vi "Save校准Spec.vi"(4 "补偿值":T3={"甩线补偿值"={"下边"=23.0, "距离上边"=10.0, "左边"=7.2, "右边"=25.8}, "补偿甩线坐标偏移"={"X"=40.0, "Y"=70.0}, "mark点补偿"={"X"=-48.38, "Y"=-84.85}, "出线补偿值"=25.8, "mark规格"={"X下限"=-48.0, "X上限"=-84.0, "Y下限"=0.0, "Y 上限"=0.0, "angle下限"=0.0, "angle上限"=0.0}} {"mark规格"."angle上限" format="%#.3f"; "mark规格"."angle下限" format="%#.3f"; "mark规格"."Y下限" format="%#.3f"; "mark规格"."X下限" format="%#.3f"; "mark点补偿"."X" format="%#.3f"; "补偿甩线坐标偏移"."X" format="%#.3f"}) -> ()   [LabVIEW 2014]
uses:
  Controls/XYPos.ctl
  Global.vi
  <vilib>/Utility/file.llb/Write To Spreadsheet File (string).vi
panel:
  out "数组":string[][](array[string])
  out "File out":path
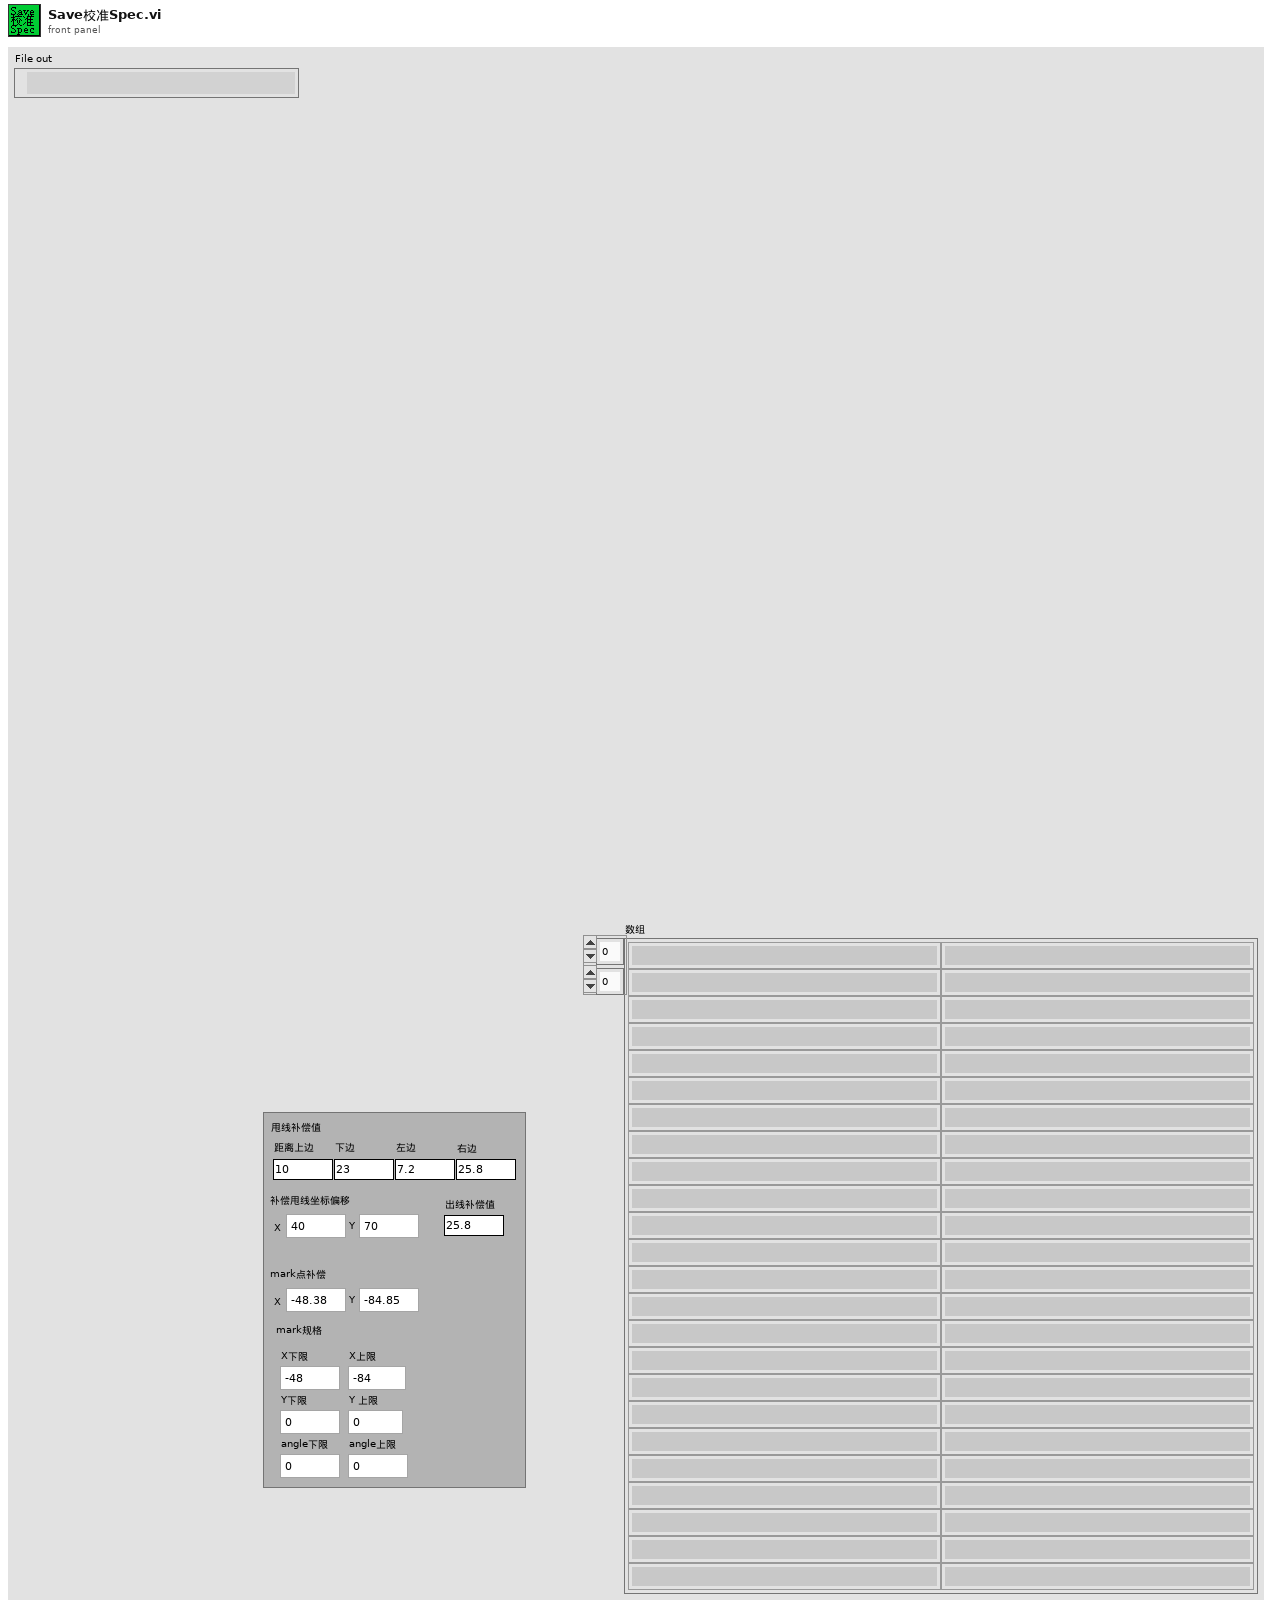
[diagram p1: front panel]
types:
  T1 = typedef "XYPos.ctl" = cluster{"X":dbl, "Y":dbl}
  T2 = typedef "mark规格.ctl" = cluster{"X下限":dbl, "X上限":dbl, "Y下限":dbl, "Y 上限":dbl, "angle下限":dbl, "angle上限":dbl}
  T3 = cluster{"甩线补偿值":cluster{"下边":dbl, "距离上边":dbl, "左边":dbl, "右边":dbl}, "补偿甩线坐标偏移":T1, "mark点补偿":T1, "出线补偿值":dbl, "mark规格":T2}
  T4 = cluster{"下边":dbl, "距离上边":dbl, "左边":dbl, "右边":dbl}
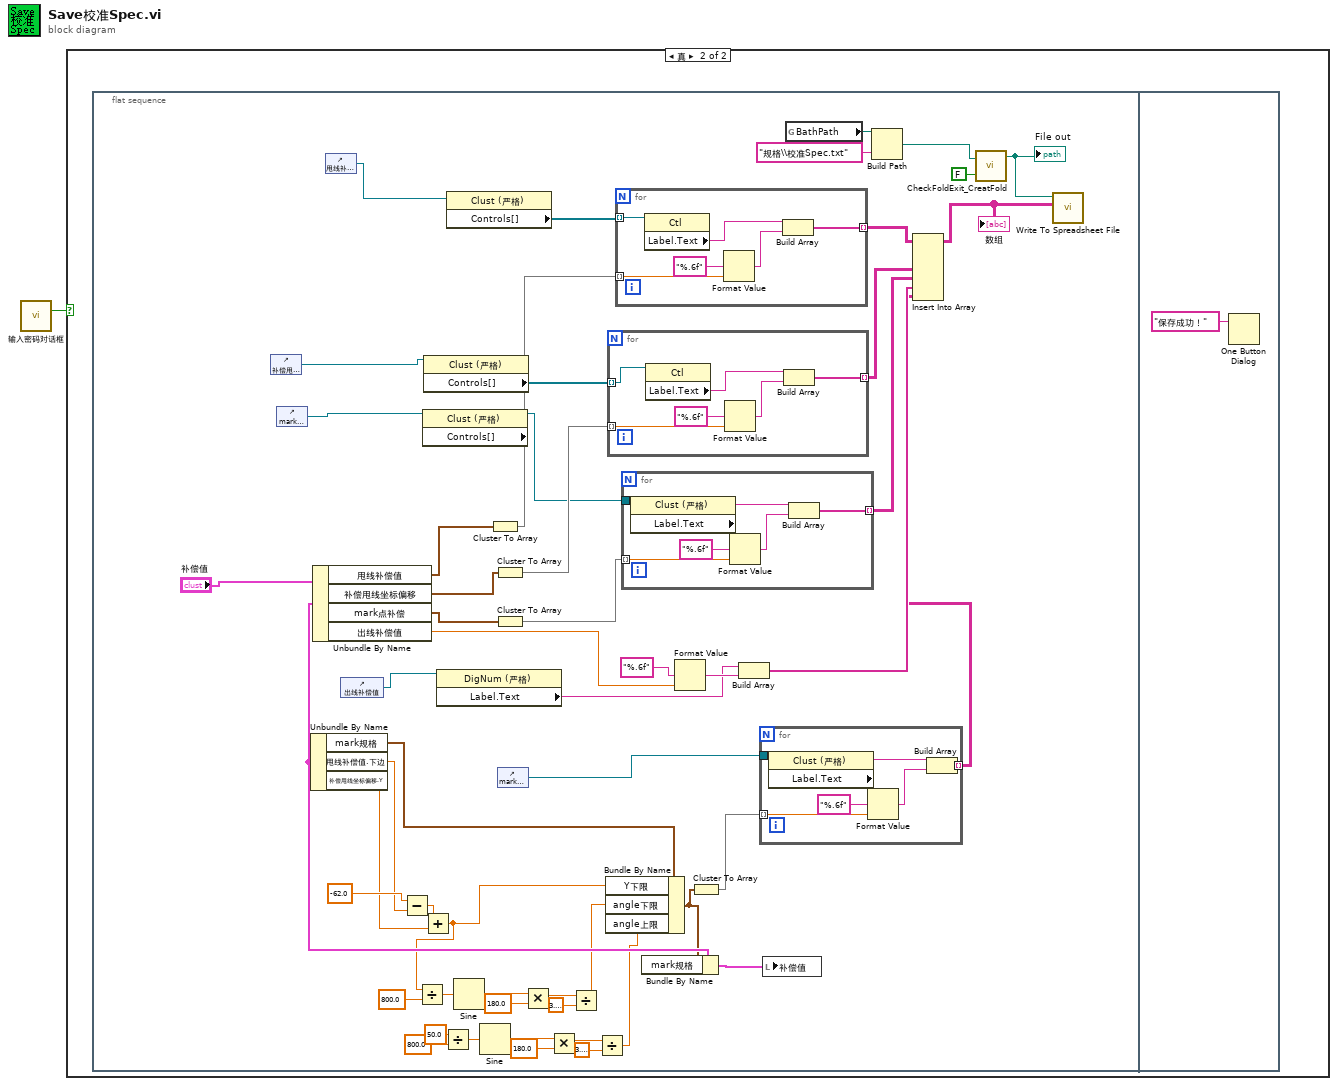
[diagram p0: block diagram]
diagram:
  n1 = call "输入密码对话框.vi"() -> ("密码正确"=w1:bool)  [unwired: 11 in]
  n2 = case shown="真" w1 {
    frame False {
    }
    frame True {
      n3 = flat-sequence {
        frame #0 {
          n4 = control-ref of="补偿甩线坐标偏移"() -> (w37:refnum<vi>)
          n5 = control-ref of="mark点补偿"() -> (w36:refnum<vi>)
          n6 = Unbundle By Name("补偿值") -> ("mark规格"=w23:T2, "甩线补偿值.下边"=w26:dbl, "补偿甩线坐标偏移.Y"=w24:dbl)
          n7 = Unbundle By Name("补偿值") -> ("甩线补偿值"=w27:T4, "补偿甩线坐标偏移"=w47:T1, "mark点补偿"=w45:T1, "出线补偿值"=w33:dbl)
          n8 = control-ref of="甩线补偿值"() -> (w38:refnum<vi>)
          n9 = control-ref of="出线补偿值"() -> (w35:refnum<vi>)
          n10 = Subtract(x=-62.0, y=w26) -> (x-y=w25:dbl)
          n11 = property class="Clust (严格)" props=["Controls[]"](reference=w36) -> (reference out=w39:refnum<vi>)  [unwired: 1 in, 2 out]
          n12 = Add(x=w25, y=w24) -> (x+y=w16:dbl)
          n13 = Divide(x=w16, y=800.0) -> (x/y=w17:dbl)
          n14 = property class="Clust (严格)"(reference=w37) -> ("Controls[]"=w40:refnum<vi>[])  [unwired: 1 in, 2 out]
          n15 = property class="DigNum (严格)"(reference=w35) -> ("Label.Text"=w30:string)  [unwired: 1 in, 2 out]
          n16 = Divide(x=50.0, y=800.0) -> (x/y=w4:dbl)
          n17 = property class="Clust (严格)"(reference=w38) -> ("Controls[]"=w50:refnum<vi>[])  [unwired: 1 in, 2 out]
          n18 = Sine(x=w17) -> (sin(x)=w14:dbl)
          n19 = Sine(x=w4) -> (sin(x)=w6:dbl)
          n20 = Cluster To Array(cluster=w27) -> (array=w48:dbl[])
          n21 = Cluster To Array(cluster=w47) -> (array=w46:dbl[])
          n22 = Cluster To Array(cluster=w45) -> (array=w44:dbl[])
          n23 = control-ref of="mark规格"() -> (w29:refnum<vi>)
          n24 = Multiply(x=w14, y=180.0) -> (x*y=w12:dbl)
          n25 = Multiply(x=w6, y=180.0) -> (x*y=w8:dbl)
          n26 = Divide(x=w12, y=3.141592653589793) -> (x/y=w10:dbl)
          n27 = Divide(x=w8, y=3.141592653589793) -> (x/y=w2:dbl)
          n28 = Bundle By Name(cluster=w23, "Y下限"=w16, "angle下限"=w10, "angle上限"=w2) -> (w19:T2)
          n29 = for {
            tunnel: [w70] -> w43 mode=indexing
            tunnel: w46 -> [w72] mode=indexing
            tunnel: w40 -> [w68] mode=indexing
            n30 = property class="Ctl"(reference=w68) -> ("Label.Text"=w69:string)  [unwired: 1 in, 2 out]
            n31 = Format Value(format string="%.6f" ("format (%.3f)"), value (0)=w72) -> (output string=w71:string)  [unwired: 1 in]
            n32 = Build Array(w69, w71) -> (w70:string[])
          }
          n33 = for {
            tunnel: [w75] -> w49 mode=indexing
            tunnel: w50 -> [w79] mode=indexing
            tunnel: w48 -> [w77] mode=indexing
            n34 = property class="Ctl"(reference=w79) -> ("Label.Text"=w74:string)  [unwired: 1 in, 2 out]
            n35 = Format Value(format string="%.6f" ("format (%.3f)"), value (0)=w77) -> (output string=w76:string)  [unwired: 1 in]
            n36 = Build Array(w74, w76) -> (w75:string[])
          }
          n37 = for {
            tunnel: [w63] -> w42 mode=indexing
            tunnel: w39 -> [w67]
            tunnel: w44 -> [w65] mode=indexing
            n38 = property class="Clust (严格)"(reference=w67) -> ("Label.Text"=w62:string)  [unwired: 1 in, 2 out]
            n39 = Format Value(format string="%.6f" ("format (%.3f)"), value (0)=w65) -> (output string=w64:string)  [unwired: 1 in]
            n40 = Build Array(w62, w64) -> (w63:string[])
          }
          n41 = Bundle By Name(cluster="补偿值", "mark规格"=w19) -> (w18:T3)
          n42 = Format Value(format string="%.6f" ("format (%.3f)"), value (0)=w33) -> (output string=w32:string)  [unwired: 1 in]
          n43 = Cluster To Array(cluster=w19) -> (array=w22:dbl[])
          n44 = Build Array(w30, w32) -> (w31:string[])
          n45 = for {
            tunnel: [w57] -> w21 mode=indexing
            tunnel: w29 -> [w61]
            tunnel: w22 -> [w59] mode=indexing
            n46 = property class="Clust (严格)"(reference=w61) -> ("Label.Text"=w56:string)  [unwired: 1 in, 2 out]
            n47 = Format Value(format string="%.6f" ("format (%.3f)"), value (0)=w59) -> (output string=w58:string)  [unwired: 1 in]
            n48 = Build Array(w56, w58) -> (w57:string[])
          }
          n49 = local write "补偿值"(w18) -> ()
          n50 = global read "Global.vi" "BathPath"() -> (w53:path)
          n51 = Build Path(base path=w53, name or relative path="规格\\校准Spec.txt" ("名称或相对路径")) -> (appended path=w52:path)
          n52 = Insert Into Array(array=w49, new element #1=w43, new element #2=w42, new element #3=w31, new element #4=w21) -> (w41:string[][])  [unwired: 2 in]
          "数组" <- w41
          n53 = call "CheckFoldExit_CreatFold.vi"("path in"=w52, "FoldOrFile¡H"=FALSE) -> ("File out"=w54:path)  [unwired: 2 out]
          "File out" <- w54
          n54 = call-poly <vilib>:"Write To Spreadsheet File.vi"("2D data"=w41, "file path (dialog if empty)"=w54) -> ()  [unwired: 6 in, 1 out]
        }
        frame #1 {
          n55 = One Button Dialog(message="保存成功！" ("消息")) -> ()  [unwired: 1 in, 1 out]
        }
      }
    }
  }
